vi "Decode Input.vi"(11 "Input":string[](array[string])) -> (3 "Data":T1)   [LabVIEW 2020]
uses:
  Data.ctl
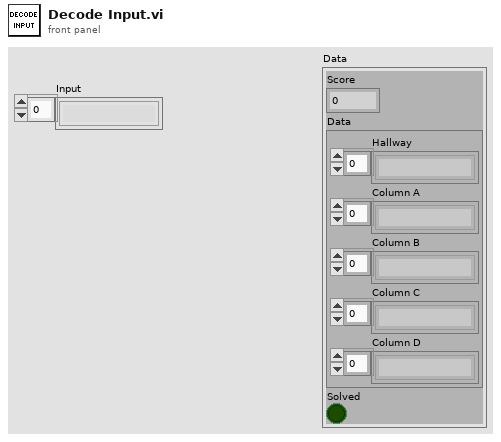
[diagram p1: front panel]
types:
  T1 = typedef "Data.ctl" = cluster{"Score":i64, "Data":cluster{"Hallway":string[], "Column A":string[], "Column B":string[], "Column C":string[], "Column D":string[]}, "Solved":bool}
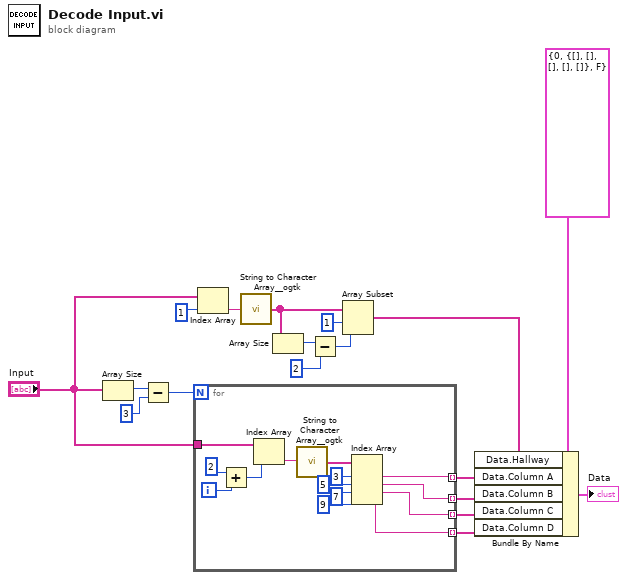
[diagram p0: block diagram]
diagram:
  n1 = Array Size(array="Input") -> (size(s)=w12:i32)
  n2 = Subtract(x=w12, y=3) -> (x-y=w14:i32)
  n3 = for {
    N: w14 -> [_]
    tunnel: "Input" -> [w32]
    tunnel: [w22] -> w18 mode=indexing
    tunnel: [w21] -> w17 mode=indexing
    tunnel: [w20] -> w16 mode=indexing
    tunnel: [w19] -> w15 mode=indexing
    i -> [w31]
    n4 = Add(x=2, y=w31) -> (x+y=w30:i32)
    n5 = Index Array(array=w32, index=w30) -> (element=w28:string)
    n6 = call <userlib>:"String to Character Array__ogtk.vi"("Input String"=w28) -> ("Character Array"=w27:string[])
    n7 = Index Array(array=w27, index #1=3 ("index"), index #2=5 ("index"), index #3=7 ("index"), index #4=9 ("index")) -> (element #1=w22:string, element #2=w21:string, element #3=w20:string, element #4=w19:string)
  }
  n8 = Index Array(array="Input", index=1) -> (element=w9:string)
  n9 = call <userlib>:"String to Character Array__ogtk.vi"("Input String"=w9) -> ("Character Array"=w7:string[])
  n10 = Array Size(array=w7) -> (size(s)=w6:i32)
  n11 = Subtract(x=w6, y=2) -> (x-y=w4:i32)
  n12 = Array Subset(array=w7, index=1, length=w4) -> (w3:string[])
  n13 = Bundle By Name(cluster=T1 {"Score"=0, "Data"={"Hallway"=[], "Column A"=[], "Column B"=[], "Column C"=[], "Column D"=[]}, "Solved"=FALSE} ("output cluster"), "Data.Hallway"=w3, "Data.Column A"=w18, "Data.Column B"=w17, "Data.Column C"=w16, "Data.Column D"=w15) -> (→"Data":T1)
